vi "Create DO Task.vi"(8 "error in":errorcluster, 11 "Line":string="cDAQ3Mod2/port0/line0") -> (0 "error out":errorcluster, 3 "task out":refnum<k21>)   [LabVIEW 2013]
uses:
  <vilib>/DAQmx/create/channels.llb/DAQmx Create Channel (DO-Digital Output).vi
  <resource>/objmgr/daqmx.rc
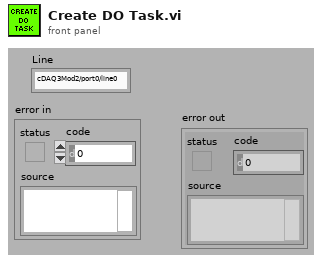
[diagram p1: front panel]
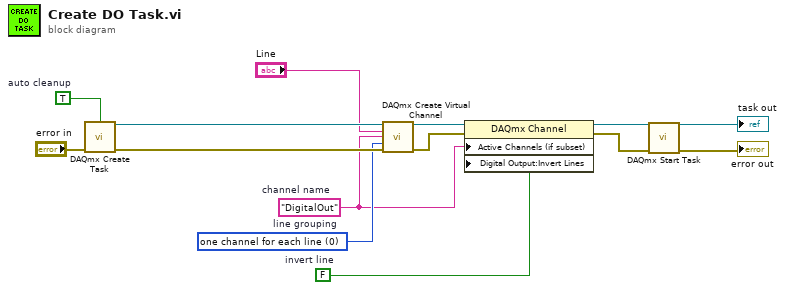
[diagram p0: block diagram]
diagram:
  w6 = FALSE  # invert line
  w9 = 0 items=["one channel for each line", "one channel for all lines"]  # line grouping
  w5 = "DigitalOut"  # channel name
  w12 = TRUE  # auto cleanup
  n1 = call <vilib>:"DAQmx Create Task.vi"("auto cleanup"=w12, "error in"="error in") -> ("task out"=w11:refnum<k21>, "error out"=w13:errorcluster)  [unwired: 12 in]
  n2 = call-poly <vilib>:"DAQmx Create Virtual Channel.vi"("task in"=w11, "lines"="Line", "name to assign"=w5, "line grouping"=w9, "error in"=w13) -> ("task out"=w8:refnum<k21>, "error out"=w7:errorcluster)  [unwired: 9 in]
  n3 = property class="DAQmx Channel"(reference=w8, error in=w7, "Active Channels (if subset)"=w5, "Digital Output:Invert Lines"=w6) -> (reference out=w4:refnum<k21>, error out=w3:errorcluster)
  n4 = call <vilib>:"DAQmx Start Task.vi"("task/channels in"=w4, "error in"=w3) -> ("task out"=→"task out":refnum<k21>, "error out"=→"error out":errorcluster)  [unwired: 12 in]
